vi "TEB StopEvent Message.vi"(0 "Event Number":i32) -> ()   [LabVIEW 2010]
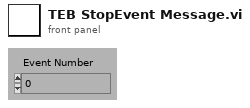
[diagram p1: front panel]
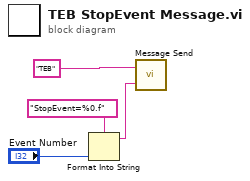
[diagram p0: block diagram]
diagram:
  n1 = Format Into String(format string="StopEvent=%0.f", "Event Number") -> (resulting string=w3:string)  [unwired: 2 in, 1 out]
  n2 = call "Message Send.vi"("Message"=w3, "Destination"="TEB" ("Destination(s)")) -> ()
